vi "Untitled 2 (SubVI).vi"(1 "x":u32, 2 "N":u32, 3 "Min":dbl, 4 "Max":dbl) -> (0 "y":dbl)   [LabVIEW 2010]
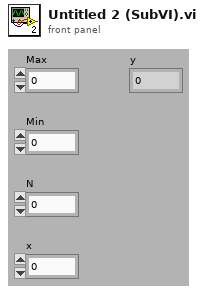
[diagram p1: front panel]
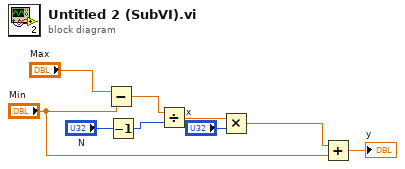
[diagram p0: block diagram]
diagram:
  n1 = Subtract(x="Max", y="Min") -> (x-y=w1:dbl)
  n2 = Decrement(x="N") -> (x-1=w2:u32)
  n3 = Divide(x=w1, y=w2) -> (x/y=w5:dbl)
  n4 = Multiply(x=w5, y="x") -> (x*y=w6:dbl)
  n5 = Add(x=w6, y="Min") -> (x+y=→"y":dbl)
